vi "Actor Core.vi"(8 "error in":errorcluster, 11 "Connecting in":refnum<class "Connecting.lvclass">) -> (0 "error out":errorcluster, 3 "Actor out":refnum<class "Actor.lvclass">)   [LabVIEW 2013, in "Receiver.lvlib" / "ReceiverStates.lvlib" / "Connecting.lvclass"]
doc: "(<B>Filename</B>: Actor Framework.lvlib:Actor.lvclass:Actor Core.vi)\n\nReceives messages to the actor, reacts to them, and initiates any error handling that may shut the actor down.\n\nDescendant classes may override this VI to append parallel tasks for the actor to complete while it handles messages. Overrides use the Call Parent Method node."
uses:
  Connecting.lvclass
  <vilib>/ActorFramework/Actor/Actor.lvclass
  ReceiverState/ReceiverState.lvclass
  ReceiverConnectedState/Connected.lvclass
  <vilib>/ni/Actors/State Actor/State Actor/State Actor.lvclass
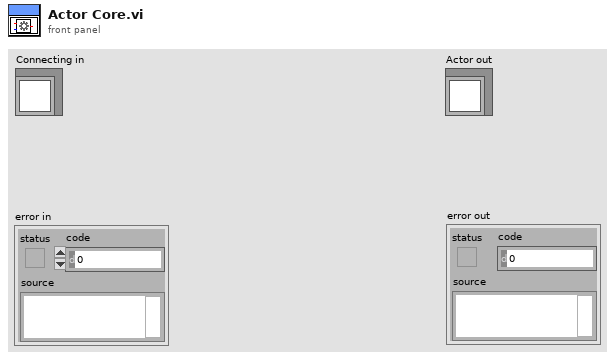
[diagram p1: front panel]
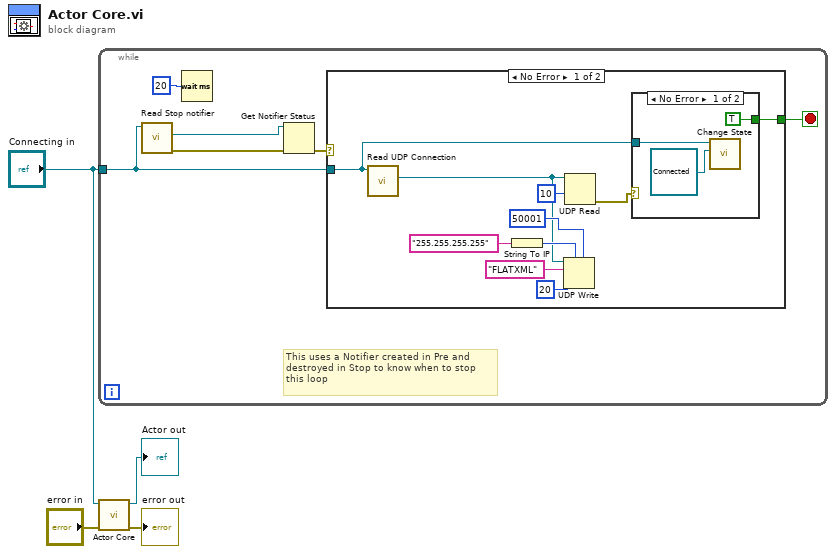
[diagram p0: block diagram]
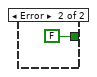
[diagram p2: hidden frame]
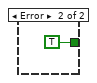
[diagram p3: hidden frame]
diagram:
  n1 = while {
    tunnel: "Connecting in" -> [w6]
    stop <- w5 stop-if-true
    # "This uses a Notifier created in Pre and\ndestroyed in Stop to know when to stop\nthis loop"
    n2 = call-dynamic "Read Stop notifier.vi"("ReceiverState in"=w6) -> ("error out"=w9:errorcluster, "Stop notifier"=w10:refnum<notifier>)  [unwired: 8 in, 1 out]
    n3 = Wait (ms)(milliseconds to wait=u32 20) -> ()  [unwired: 1 out]
    n4 = Get Notifier Status(notifier=w10, error in (no error)=w9) -> (error out=w7:errorcluster)  [unwired: 4 out]
    n5 = case shown="No Error" w7 {
      tunnel: w6 -> [w13 _]
      tunnel: [w14 TRUE] -> w5
      frame No Error {
        n6 = call-dynamic "Read UDP Connection .vi"("ReceiverState in"=w13) -> ("UDP Connection"=w16:refnum<k16>)  [unwired: 8 in, 2 out]
        n7 = String To IP(1:"255.255.255.255") -> (0:w20:u32)
        n8 = UDP Write(address=w20, port or service name=u32 50001 ("address"), connection ID=w16, data in="FLATXML", 9:20 ("timeout ms (25000)")) -> ()  [unwired: 1 in, 2 out]
        n9 = UDP Read(connection ID=w16, timeout ms (25000)=10) -> (error out=w15:errorcluster)  [unwired: 2 in, 4 out]
        n10 = case shown="No Error" w15 {
          tunnel: [TRUE FALSE] -> w14
          tunnel: w13 -> [w21 _]
          frame No Error {
            n11 = call <vilib>:"Change State.vi"("New State in"=refnum<class "Connected.lvclass"> refnum ("Receiver.lvlib:ReceiverStates.lvlib:Connected.lvclass"), "State in"=w21) -> ()  [unwired: 8 in, 2 out]
          }
          frame Error {
          }
        }
      }
      frame Error {
      }
    }
  }
  n12 = call-parent "Actor Core.vi"("error in"="error in", "ReceiverState in"="Connecting in") -> ("error out"=→"error out":errorcluster, "Actor out"=→"Actor out":refnum<class "Actor.lvclass">)  [unwired: 8 in]
